vi "demo_Windows Long Path Support.vi"(11 "Stop Demo":refnum<user-event>) -> ()   [LabVIEW 2020]
panel:
  in  "Long Path":path=path "C:/Folder 1/Folder 2/Folder 3/Folder 4/Folder 5/Folder 6/Folder 7/Folder 8/Folder 9/Folder 10/Folder 11/Folder 12/Folder 13/Folder 14/Folder 15/Folder 16/Folder 17/Folder 18/Folder 19/Folder 20/Folder 21/Folder 22/Folder 23/Folder 24/Folder 25/Folder 26/Folder 27/Folder 28/Folder 29/Folder 30/Folder BaskinRobbins"
  # "LabVIEW 2025 Q3 - Windows Long Path Support\n\nWindows long paths (paths with a number of characters exceeding 250) are  supported by all parts of LabVIEW, including the file loading system and App Builder."
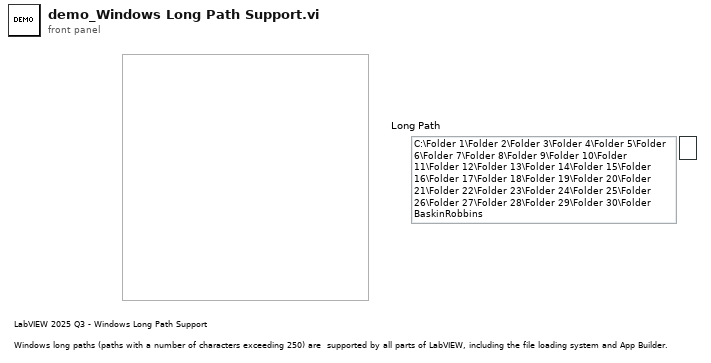
[diagram p1: front panel]
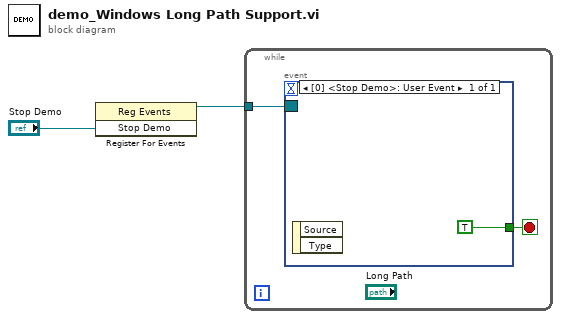
[diagram p0: block diagram]
diagram:
  n1 = register-events("Stop Demo") -> (reference out=w1:refnum<event-registration>)  [unwired: 2 in, 1 out]
  n2 = while {
    tunnel: w1 -> [w4]
    stop <- w3 stop-if-true
    n3 = event shown="[0] <Stop Demo>: User Event" {
      selector: w4 -> [_]
      dyn-events: _ -> [_]
      timeout: _ -> [_]
      tunnel: [TRUE] -> w3
      event User Event {
        n4 = event-data() -> ()  [unwired: 1 in, 2 out]
      }
    }
  }
